vi "TestExec.Health Status, Set Error_Warning.vi"(7 "Module Q Name":string, 8 "error in":errorcluster, 10 "Health State Cmd":T1=enum."Set Warning", 11 "Q In":refnum<queue>) -> (0 "error out":errorcluster)   [LabVIEW 2018]
uses:
  <vilib>/KATE/Queues/Q.Element.ctl
  TestExec.Health State Command.ctl
  <vilib>/KATE/Queues/Queue Utils.lvlib
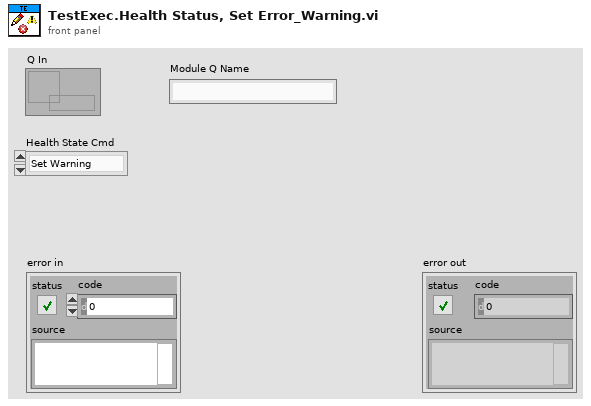
[diagram p1: front panel]
types:
  T1 = typedef "TestExec.Health State Command.ctl" = enum16{"Update", "Clear All", "Clear Warnings", "Clear Errors", "Set Warning", "Set Error"}
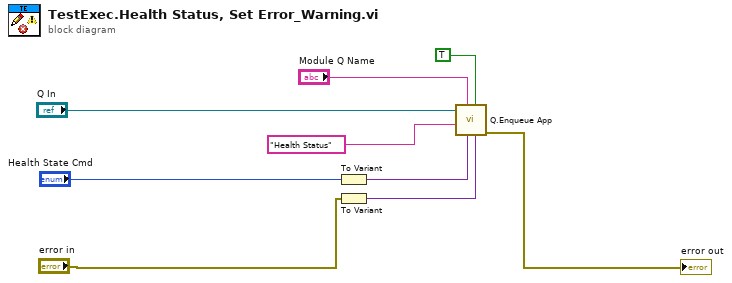
[diagram p0: block diagram]
diagram:
  n1 = To Variant(anything="Health State Cmd") -> (Variant=w4:variant)
  n2 = To Variant(anything="error in") -> (Variant=w1:variant)
  n3 = call <vilib>:"Q.Enqueue App.vi"("Data2"=w1, "Top of Q"=TRUE, "Data1"=w4, "Q Name"="Module Q Name", "Task Name"="Health Status" ("Cmd"), "Q In"="Q In") -> ("error out"=→"error out":errorcluster)  [unwired: 4 in, 1 out]
